vi "Approach with PicoMotors.vi"(7 "Computer called (T/F)":bool) -> ()   [LabVIEW 2023]
uses:
  Sub_Vi/TypeDefs/WayPointCluster.ctl
  Sub_Vi/TypeDefs/Settings.ctl
  Sub_Vi/TypeDefs/ChangeOnFly.ctl
  Sub_Vi/TypeDefs/Display.ctl
  Sub_Vi/TypeDefsControls/Feedback Type.ctl
  Settings.vi
panel:
  in  "vi path":path
  in  "Feedback Type":T1
  in  "Display Cluster":T2
  in  "ChangeonFly":T3
  in  "SettingsCluster":T4={"Sample Rate (us)"=1, "Samples Per Data Point (int, power of 2)"=1000, "DistanceToBulk (um)"=-1.0, "HoldTimeScaler"=0, "SaveData"=TRUE, "DistanceToBulk (um) 2"=-1.0, "DistanceToBulk (um) 3"=-1.0}
  in  "WayPointCluster":T5
  in  "Tab Control":T6(tab)
  out "Current 1":cluster{"Y":dbl[], "Y":dbl[]}[](graph)
  out "Current 4":cluster{"Y":dbl[], "Y":dbl[]}[](graph)
  out "Current 5":cluster{"Y":dbl[], "Y":dbl[]}[](graph)
  out "Current 6":dbl[](graph)
  out "Current 2":dbl[](graph)
  out "Current 3":dbl[](graph)
  in  "Feedback Threshold":dbl=1e-13
  in  "Greater Than":bool=TRUE
  in  "Retract Piezo after approach (T/F)":bool=TRUE
  in  "Approach Voltage (V)":dbl=0.35 min=-5.0 max=5.0
  in  "Approach Rate (µm/s)":dbl=0.1 min=0.0 max=38.0
  in  "End Extension (µm)":dbl=38.0 min=0.0 max=100.0
  in  "Start Extention (µm)":dbl min=0.0 max=100.0
  in  "Start scan Button":bool
  in  "stop 2":bool
  in  "Pause":bool
  out "Phase":dbl[](graph)
  out "Amplitude":dbl[](graph)
  # "Settings"
  # "Pause at"
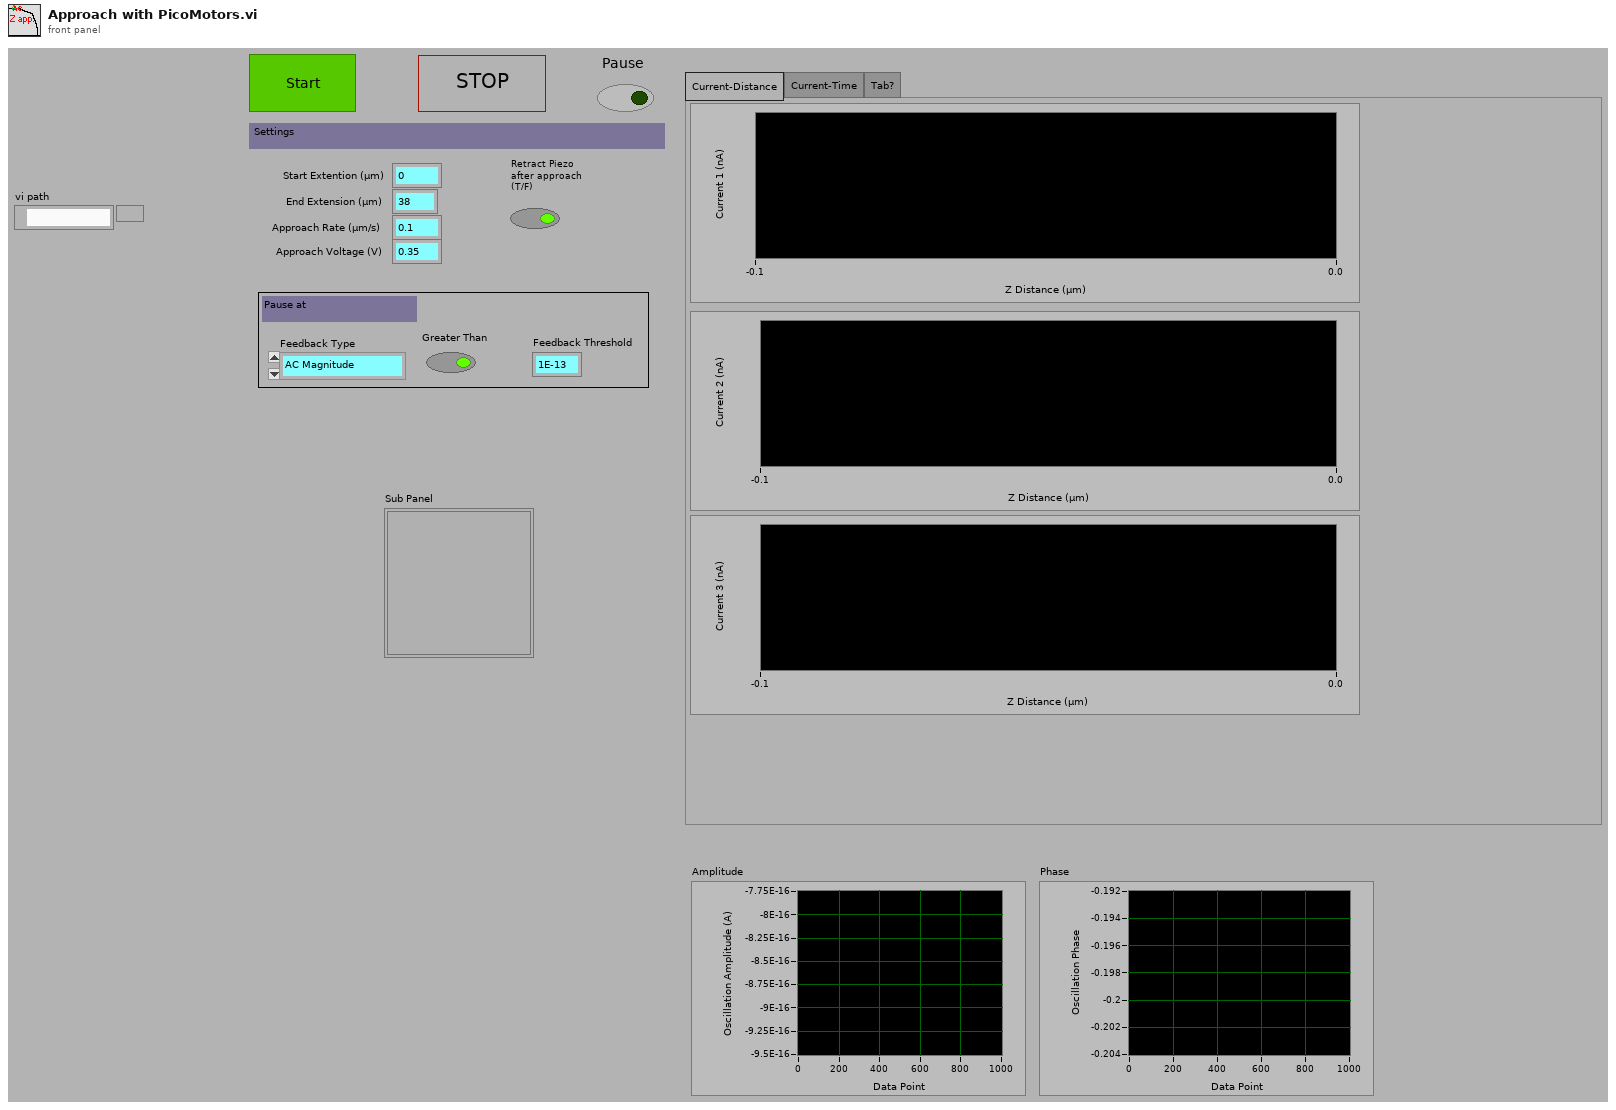
[diagram p1: front panel]
types:
  T1 = typedef "Feedback Type.ctl" = enum16{"AC Magnitude", "Current 1", "Current 2", "Phase"}
  T2 = typedef "Display.ctl" = cluster{"X":refnum<vi>, "Y":refnum<vi>, "Z":refnum<vi>, "Amp":refnum<vi>, "Phase":refnum<vi>, "t vs Z":refnum<vi>, "t vs C1":refnum<vi>, "t vs C2":refnum<vi>, "t vs C3":refnum<vi>, "t vs Amp":refnum<vi>, "t vs Phase":refnum<vi>, "t vs X":refnum<vi>, "t vs Y":refnum<vi>, "Z vs C1":refnum<vi>, "Z vs C2":refnum<vi>, "Z vs C3":refnum<vi>, "V vs C1":refnum<vi>, "V vs C2":refnum<vi>, "V vs C3":refnum<vi>, "X/Y/Z F":refnum<vi>, "X/Y/Z R":refnum<vi>, "X/Y/C1 F":refnum<vi>, "X/Y/C1 R":refnum<vi>, "X/Y/C2 F":refnum<vi>, "X/Y/C2 R":refnum<vi>, "X/Y/C3 F":refnum<vi>, "X/Y/C3 R":refnum<vi>, "NumberOfLines":u16, "um Per Pixel":dbl, "um Per Line":dbl, "X Center":dbl, "Hop X/Y/Z":refnum<vi>, "Hop X/Y/C1":refnum<vi>, "Hop X/Y/C2":refnum<vi>, "Hop X/Y/C3":refnum<vi>, "X Width":dbl, "Y Width":dbl, "Hopping Distance":dbl, "V2 vs C1":refnum<vi>, "V vs Phase":refnum<vi>, "Y Center":dbl, "Number of Pixels":dbl, "V2 vs C2":refnum<vi>, "V2 vs C3":refnum<vi>, "V vs y":refnum<vi>, "V2 vs y":refnum<vi>, "Z vs Amp":refnum<vi>, "Z vs Phase":refnum<vi>}
  T3 = typedef "ChangeOnFly.ctl" = cluster{"Stop (boolean)":refnum<vi>, "Pause (boolean)":refnum<vi>, "EndCurrentLine (boolean)":refnum<vi>, "max movement per update step (Interger, nm)":refnum<vi>, "P (float, arb)":refnum<vi>, "Feedback set point (double, Amps)":refnum<vi>, "Voltage (double, V)":refnum<vi>, "Feedback set point 2 (double, Amps)":refnum<vi>, "Stop on Greater Than 2? (boolean)":refnum<vi>, "Stop on Greater Than? (boolean)":refnum<vi>, "Voltage 2 (double, V)":refnum<vi>, "Feedback Type (enum)":refnum<vi>, "Feedback Type 2 (enum)":refnum<vi>}
  T4 = typedef "Settings.ctl" = cluster{"Sample Rate (us)":u32, "Samples Per Data Point (int, power of 2)":i16, "DistanceToBulk (um)":dbl, "HoldTimeScaler":u64, "SaveData":bool, "DistanceToBulk (um) 2":dbl, "DistanceToBulk (um) 3":dbl}
  T5 = typedef "WayPointCluster.ctl" = cluster{"X (um)":dbl[], "Y (um)":dbl[], "Z (um)":dbl[], "V (V)":dbl[], "X Velocity (um s-1)":dbl[], "Y Velocity (um s-1)":dbl[], "Z Velocity (um s-1)":dbl[], "V Velocity (V s-1)":dbl[], "FeedBack Type (enum)":u16[], "Move X (boolean)":bool[], "Move Y (boolean)":bool[], "Move Z (boolean)":bool[], "Move V (boolean)":bool[], "Jump V (boolean)":bool[], "Hold (boolean)":bool[], "Hold Time":u32[], "V2 (V)":dbl[], "Move V2":bool[], "V2 Velocity (V s-1)":dbl[], "Jump V2 (boolean)":bool[], "Update z Position delta (ms)":i16[], "Hold Feedback1":bool[], "Move Z PicoMotor":bool[], " Z PicoMotor Direction":bool[], "DIO0":bool[]}
  T6 = enum32{"Current-Distance", "Current-Time", "Tab?"}
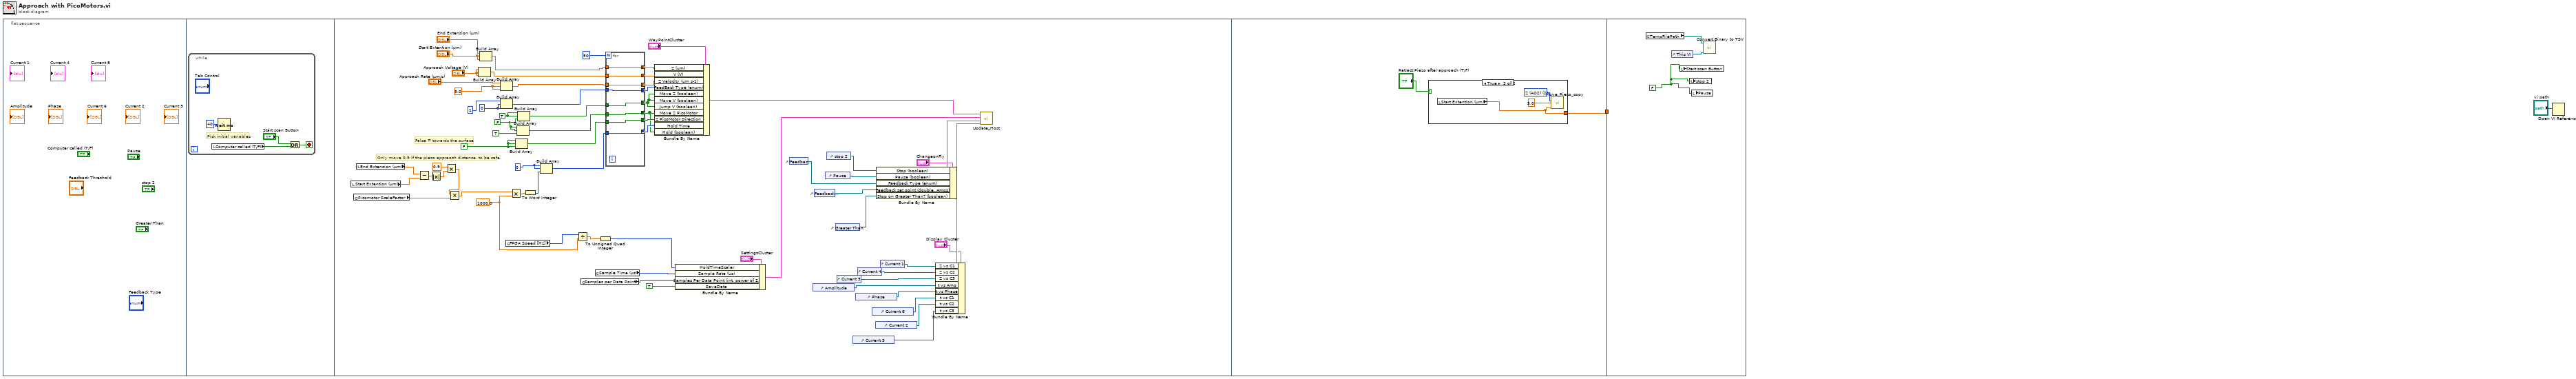
[diagram p0: block diagram]
diagram:
  n1 = flat-sequence {
    tunnel: [w82] -> w2
    tunnel: w2 -> [_]
    frame #0 {
    }
    frame #1 {
      n2 = while {
        stop <- w6 stop-if-true
        # "Pick initial variables"
        n3 = local read "Computer called (T/F)"() -> (w4:bool)
        n4 = Wait (ms)(milliseconds to wait=u32 40) -> ()  [unwired: 1 out]
        n5 = Or(x="Start scan Button", y=w4) -> (x .or. y?=w6:bool)
      }
    }
    frame #2 {
      w43 = FALSE ("Direction\n (on = positive, off = negative)")
      w8 = 1000.0
      w25 = 5.0 ("element")
      w42 = u32 0
      w45 = FALSE ("Save Data")
      w47 = u16 0
      w46 = TRUE ("Save Data")
      # "Only move 0.9 if the piezo appraoch distance, to be safe."
      # "False = towards the surface"
      n6 = local read "Start Extention (µm)"() -> (w22:dbl)
      n7 = global read "Settings.vi" "Picomotor ScaleFactor"() -> (w16:dbl)
      n8 = local read "End Extension (µm)"() -> (w23:dbl)
      n9 = Subtract(x=w23, y=w22) -> (x-y=w21:dbl)
      n10 = Absolute Value(x=w21) -> (abs(x)=w20:dbl)
      n11 = Multiply(x=0.9, y=w20) -> (x*y=w18:dbl)
      n12 = Multiply(x=w18, y=w16) -> (x*y=w41:dbl)
      n13 = Build Array("Approach Voltage (V)", "Approach Voltage (V)", "Approach Voltage (V)") -> (w38:dbl[])
      n14 = Build Array("End Extension (µm)", "Start Extention (µm)", "Start Extention (µm)") -> (w40:dbl[])
      n15 = Build Array("Approach Rate (µm/s)", w25, w25) -> (w36:dbl[])
      n16 = Build Array(u16 1, w47, w47) -> (w34:u16[])
      n17 = global read "Settings.vi" "FPGA Speed [Hz]"() -> (w15:i64)
      n18 = Multiply(x=w41, y=w8) -> (x*y=w12:dbl)
      n19 = Build Array(w43, w43, w43) -> (w31:bool[])
      n20 = Build Array(w45, w45, TRUE ("Save Data")) -> (w32:bool[])
      n21 = Build Array(w46, w46, w45) -> (w33:bool[])
      n22 = To Word Integer(number=w12) -> (16bit integer=w11:i16)
      n23 = Build Array(w42, w42, w11) -> (w30:u32[])
      n24 = Divide(x=w15, y=w8) -> (x/y=w14:dbl)
      n25 = global read "Settings.vi" "Samples per Data Point"() -> (w53:u16)
      n26 = global read "Settings.vi" "Sample Time (µs)"() -> (w54:u32)
      n27 = To Unsigned Quad Integer(1:w14) -> (0:w13:u64)
      n28 = for {
        N: 50 -> [_]
        tunnel: w40 -> [w81]
        tunnel: [w81] -> w39 mode=concatenating
        tunnel: w38 -> [w80]
        tunnel: [w80] -> w37 mode=concatenating
        tunnel: w36 -> [w79]
        tunnel: [w79] -> w35 mode=concatenating
        tunnel: w34 -> [w78]
        tunnel: [w78] -> w27 mode=concatenating
        tunnel: w33 -> [w74]
        tunnel: w32 -> [w75]
        tunnel: w31 -> [w76]
        tunnel: w30 -> [w77]
        tunnel: [w77] -> w29 mode=concatenating
        tunnel: [w76] -> w10 mode=concatenating
        tunnel: [w75] -> w9 mode=concatenating
        tunnel: [w74] -> w28 mode=concatenating
      }
      n29 = Bundle By Name(cluster="WayPointCluster", "Z (um)"=w39, "V (V)"=w37, "Z Velocity (um s-1)"=w35, "FeedBack Type (enum)"=w27, "Move Z (boolean)"=w28, "Move V (boolean)"=w28, "Jump V (boolean)"=w28, "Move Z PicoMotor"=w9, "Z PicoMotor Direction"=w10, "Hold Time"=w29, "Hold (boolean)"=w9) -> (w71:T5)
      n30 = Bundle By Name(cluster="SettingsCluster", "HoldTimeScaler"=w13, "Sample Rate (us)"=w54, "Samples Per Data Point (int, power of 2)"=w53, "SaveData"=TRUE ("Save Data")) -> (w69:T4)
      n31 = control-ref of="Feedback Type"() -> (w17:refnum<vi>)
      n32 = control-ref of="Amplitude"() -> (w62:refnum<vi>)
      n33 = control-ref of="Feedback Threshold"() -> (w67:refnum<vi>)
      n34 = control-ref of="Pause"() -> (w65:refnum<vi>)
      n35 = control-ref of="stop 2"() -> (w66:refnum<vi>)
      n36 = control-ref of="Greater Than"() -> (w24:refnum<vi>)
      n37 = control-ref of="Current 5"() -> (w64:refnum<vi>)
      n38 = control-ref of="Current 3"() -> (w58:refnum<vi>)
      n39 = control-ref of="Phase"() -> (w61:refnum<vi>)
      n40 = control-ref of="Current 4"() -> (w63:refnum<vi>)
      n41 = control-ref of="Current 6"() -> (w60:refnum<vi>)
      n42 = control-ref of="Current 2"() -> (w59:refnum<vi>)
      n43 = Bundle By Name(cluster="ChangeonFly", "Stop (boolean)"=w66, "Pause (boolean)"=w65, "Feedback Type (enum)"=w17, "Feedback set point (double, Amps)"=w67, "Stop on Greater Than? (boolean)"=w24) -> (w68:T3)
      n44 = control-ref of="Current 1"() -> (w72:refnum<vi>)
      n45 = Bundle By Name(cluster="Display Cluster", "Z vs C1"=w72, "Z vs C2"=w63, "Z vs C3"=w64, "t vs Amp"=w62, "t vs Phase"=w61, "t vs C1"=w60, "t vs C2"=w59, "t vs C3"=w58) -> (w70:T2)
      n46 = call "Update_Host.vi"("Display Cluster"=w70, "ChangeonFly"=w68, "SettingsCluster"=w69, "WayPointCluster"=w71) -> ()  [unwired: 6 in]
    }
    frame #3 {
      n47 = case shown="True" "Retract Piezo after approach (T/F)" {
        tunnel: [_ w84] -> w82
        frame False {
        }
        frame True {
          w86 = u16 2 items=["X (AO0)", "Y (AO1)", "Z (AO2)", "V (AO3)"] ("Channel")
          n48 = local read "Start Extention (µm)"() -> (w84:dbl)
          n49 = call "Move_Piezo_copy.vi"("Piezo"=w86, "Movement Speed (µm/s)"=5.0 ("Scan Rate (um/s)"), "Position (µm) (or V)"=w84) -> ()  [unwired: 13 in]
        }
      }
    }
    frame #4 {
      w89 = FALSE ("stop recording")
      n50 = global read "Settings.vi" "TempFilePath"() -> (w87:path)
      n51 = control-ref of="This VI"() -> (w88:refnum<vi>)
      n52 = local write "Start scan Button"(w89) -> ()
      n53 = local write "stop 2"(w89) -> ()
      n54 = local write "Pause"(w89) -> ()
      n55 = call "Convert Binary to TSV.vi"("This VI"=w88, "TDMS DataFile Name"=w87) -> ()  [unwired: 10 in]
    }
  }
  n56 = Open VI Reference(vi path="vi path") -> ()  [unwired: 5 in, 2 out]
